vi "feedback node.vi"() -> ()   [LabVIEW 2012]
panel:
  out "X+Y":dbl
  in  "Boolean":bool
  in  "stop":bool
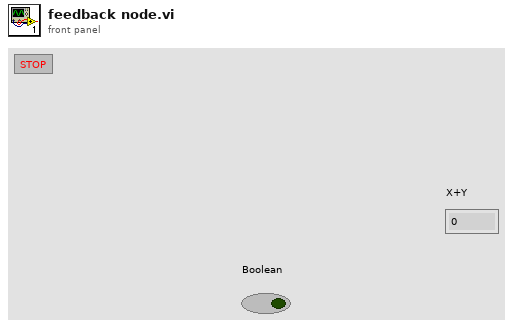
[diagram p1: front panel]
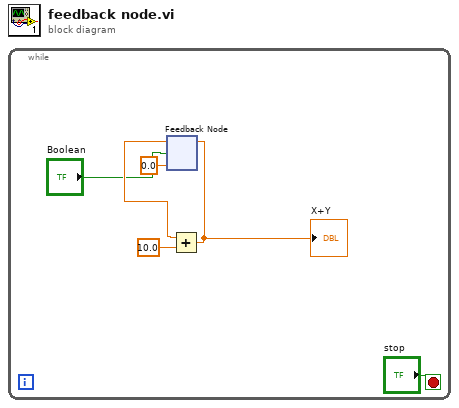
[diagram p0: block diagram]
diagram:
  n1 = while {
    stop <- "stop" stop-if-true
    n2 = feedback #1(0.0) -> (w3:dbl)
    n3 = Add(x=w3, y=10.0) -> (x+y=w4:dbl)
    "X+Y" <- w4
    n4 = feedback-in #1(w4, "Boolean") -> ()
  }
